vi "Test-Elevator-Set Percent.vi"() -> ()   [LabVIEW 2014, in "Comp Elevator.lvlib"]
uses:
  Comp Elevator.lvlib
  Robot Actor Framework/Trace/Trace Controller Class/Config.ctl
  Comp Motors with Encoders/Comp Motors with Encoders Class/Motor Controller Config.ctl
  Robot/Motor with Encoders/Motors with Encoders Class/Motors with Encoders Config.ctl
  Comp Motors with Encoders/Comp Motors with Encoders Class/Encoder Config.ctl
  Robot/Elevator/Elevator Class/Elevator Config.ctl
  Robot/Motor with Encoders/Motors with Encoders Class/Motors with Encoders.lvclass
  Comp Motors with Brake/Comp Motors with Brake Class/Comp Motors with Brake Config.ctl
  <vilib>/Rock Robotics/WPI/Solenoid/WPI_SolenoidChannel.ctl
  Comp Trace Controller/Comp Trace Controller Class/Comp Trace Controller.lvclass
  Comp Pressure/Comp Pressure Class/Comp Pressure.lvclass
  Robot/Elevator/Elevator Class/Elevator.lvclass
  Comp Motors with Brake/Comp Motors with Brake Class/Comp Motors with Brake.lvclass
  <vilib>/Rock Robotics/WPI/DriverStation/WPI_DriverStationRobotMode2.ctl
  Robot/Elevator/Elevator Messages/Set Rate (Percent) Msg/Set Rate (Percent) Msg.lvclass/Set Rate (Percent) Msg.ctl
  <vilib>/ActorFramework/Message Enqueuer/Message Enqueuer.lvclass/Message Enqueuer.ctl
  <vilib>/ActorFramework/Message Enqueuer/Enqueue.vi
  <vilib>/ActorFramework/Message Priority Queue/Priority Enqueue.vi
  Robot/Elevator/Elevator Messages/Set Rate (Percent) Msg/Set Rate (Percent) Msg.lvclass
  <vilib>/ActorFramework/Stop Msg/Stop Msg.lvclass
  <vilib>/ActorFramework/Actor/Actor.lvclass
  Robot Actor Framework/Trace/Trace Controller Class/Trace Controller.lvclass
  Comp Motors with Encoders/Comp Motors with Encoders Class/Comp Motors with Encoders.lvclass
panel:
  in  "Comp Motors with Brake Config":T1={"Brake Channel"=enum."Solenoid 6", "Pneumatics CAN ID"=3}
  in  "Radio Buttons":enum32{"Up", "Hold", "Down"}(radio)
  in  "Elevator Config":T3
  in  "Test Loop":u32=75
  in  "Encoder Config":T4={"P"=1.0, "D"=0.0, "F"=0.01, "I"=0.01, "Reverse Feedback Sensor"=FALSE, "Encoder Codes Per Rev"=256}
  out "Enable Tele":bool caption="Enabled Teleop"
  in  "Stop Test Loop 1":bool=TRUE
  in  "Finish Test":bool=TRUE
  in  "Start Test":bool=TRUE
  in  "Rate (Percent)":dbl(slide)=0.040816326530612165 scale=-1.0..1.0
  in  "Motos with Encoder Config":T5={"Counts  Per Revolution"=256, "Invert Encoder Direction"=FALSE, "Diameter of Revolution"=6.0, "Max RPM"=1500.0, "Encoder Control"=TRUE}
  in  "Slave Motor Controller Configs":T6[](array[typedef])
  in  "Master Motor Controller Config":T6={"Device Number"=7, "Invert Motor"=FALSE}
  in  "Trace Controller Config":T7={"Folder Pattern"="/media/sd%s1", "Starting Letter Position"=1, "Min Free Space (MB)"=50.0, "Max Folders to Check"=10, "Trace Level"=enum."Debug"} {"Min Free Space (MB)" format="%#_13g"}
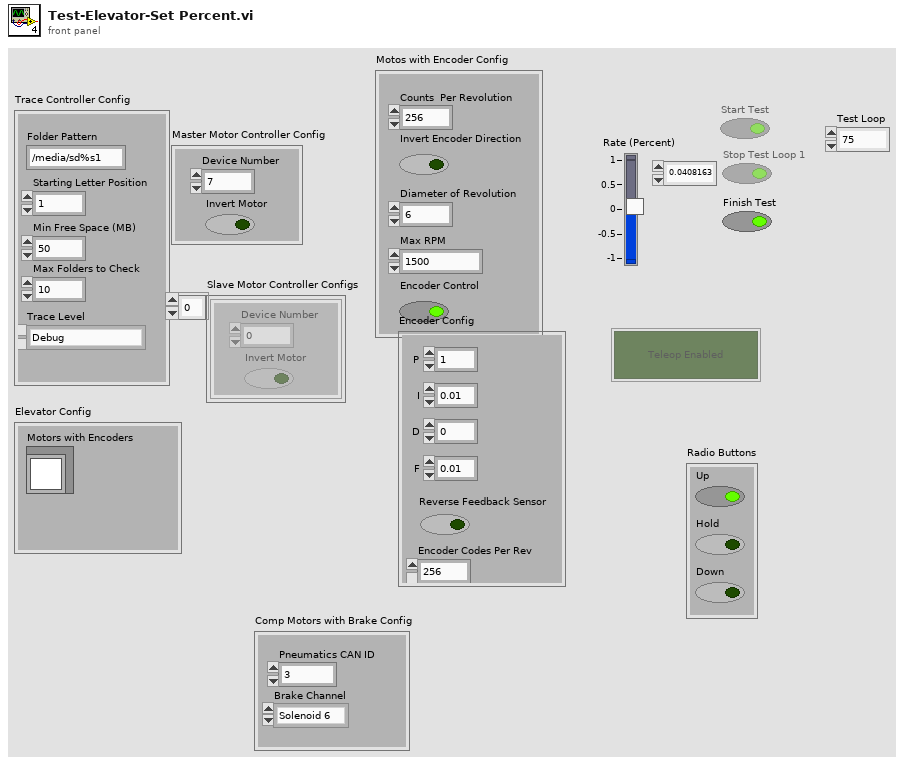
[diagram p1: front panel]
types:
  T1 = typedef "Comp Motors with Brake.lvlib/Comp Motors with Brake.lvclass/Comp Motors with Brake Config.ctl" = cluster{"Brake Channel":T2, "Pneumatics CAN ID":u8}
  T2 = typedef "WPI_SolenoidChannel.ctl" = enum8{"Solenoid 0", "Solenoid 1", "Solenoid 2", "Solenoid 3", "Solenoid 4", "Solenoid 5", "Solenoid 6", "Solenoid 7", "Invalid"}
  T3 = typedef "Elevator.lvlib/Elevator.lvclass/Elevator Config.ctl" = cluster{"Motors with Encoders ":refnum<class "Motors with Encoders.lvclass">}
  T4 = typedef "Comp Motors with Encoders.lvlib/Comp Motors with Encoders.lvclass/Encoder Config.ctl" = cluster{"P":dbl, "D":dbl, "F":dbl, "I":dbl, "Reverse Feedback Sensor":bool, "Encoder Codes Per Rev":u16}
  T5 = typedef "Motors with Encoders.lvlib/Motors with Encoders.lvclass/Motors with Encoders Config.ctl" = cluster{"Counts  Per Revolution":u32, "Invert Encoder Direction":bool, "Diameter of Revolution":dbl, "Max RPM":dbl, "Encoder Control":bool}
  T6 = typedef "Comp Motors with Encoders.lvlib/Comp Motors with Encoders.lvclass/Motor Controller Config.ctl" = cluster{"Device Number":u8, "Invert Motor":bool}
  T7 = typedef "Robot Actor Framework.lvlib/Trace.lvlib/Trace Controller.lvclass/Config.ctl" = cluster{"Folder Pattern":string, "Starting Letter Position":i32, "Min Free Space (MB)":dbl, "Max Folders to Check":u32, "Trace Level":enum16{"Critical", "Error", "Warning", "Informational", "Debug"}}
  T8 = enum16{"Critical", "Error", "Warning", "Informational", "Debug"}
  T9 = enum8{"Enabled", "Disabled", "Disabled and Grayed Out"}
  T10 = typedef "WPI_DriverStationRobotMode2.ctl" = enum16{"Autonomous Disabled", "Autonomous Enabled", "Teleop Disabled", "Teleop Enabled", "Disconnected", "Finish", "Test Disabled", "Test Enabled", "Emergency Stopped"}
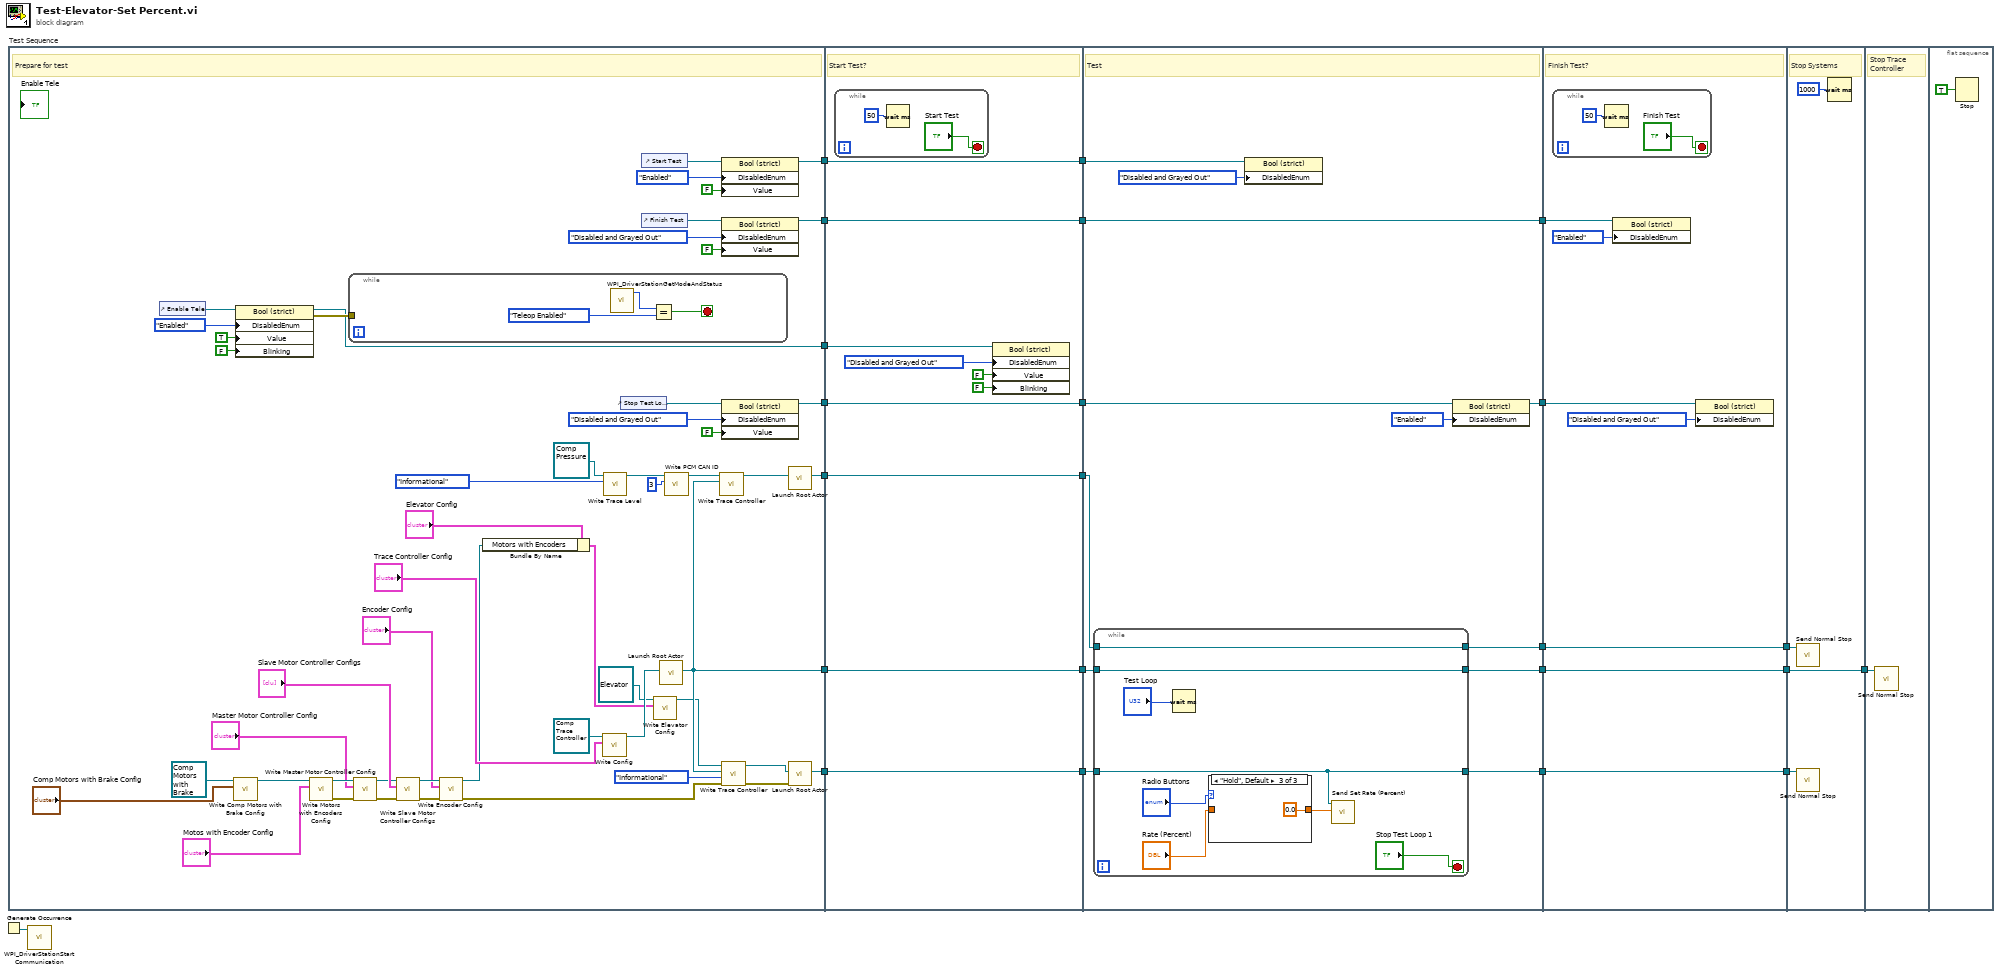
[diagram p0: block diagram]
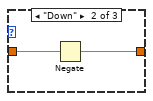
[diagram p3: hidden frame]
diagram:
  n1 = Generate Occurrence() -> (w23:refnum<k4>)
  n2 = flat-sequence "Test Sequence" {
    tunnel: [w58] -> w12
    tunnel: [w60] -> w11
    tunnel: [w59] -> w10
    tunnel: [w48] -> w9
    tunnel: [w47] -> w7
    tunnel: [w46] -> w2
    tunnel: [w40] -> w1
    tunnel: [w88] -> w15
    tunnel: [w87] -> w14
    tunnel: [w86] -> w13
    tunnel: w12 -> [w88]
    tunnel: w11 -> [w87]
    tunnel: w10 -> [w86]
    tunnel: w9 -> [w85]
    tunnel: [w85] -> w8
    tunnel: w7 -> [w84]
    tunnel: [w84] -> w6
    tunnel: [w83] -> w3
    tunnel: w2 -> [w83]
    tunnel: w1 -> [w82]
    tunnel: [w97] -> w18
    tunnel: [w99] -> w17
    tunnel: [w98] -> w16
    tunnel: w15 -> [w102]
    tunnel: w14 -> [w100]
    tunnel: w13 -> [w101]
    tunnel: w8 -> [w96]
    tunnel: w6 -> [w94]
    tunnel: [w92] -> w5
    tunnel: [w91] -> w4
    tunnel: w3 -> [w91]
    tunnel: [w121] -> w21
    tunnel: [w120] -> w20
    tunnel: [w119] -> w19
    tunnel: w18 -> [w121]
    tunnel: w17 -> [w120]
    tunnel: w16 -> [w119]
    tunnel: w5 -> [w118]
    tunnel: w4 -> [w115]
    tunnel: [w127] -> w22
    tunnel: w21 -> [w127]
    tunnel: w20 -> [w126]
    tunnel: w19 -> [w124]
    tunnel: w22 -> [w128]
    frame #0 {
      # "Prepare for test"
      n3 = control-ref of="Enable Tele"() -> (w45:refnum<vi>)
      n4 = call-dynamic "Write Comp Motors with Brake Config.vi"("Comp Motors with Brake Config"="Comp Motors with Brake Config", "Comp Motors with Brake in"=refnum<class "Comp Motors with Brake.lvclass"> refnum ("Comp Motors with Brake.lvlib:Comp Motors with Brake.lvclass")) -> ("Comp Motors with Brake out"=w25:refnum<class "Comp Motors with Brake.lvclass">)  [unwired: 8 in, 1 out]
      n5 = property class="Bool (strict)"(reference=w45, "DisabledEnum"=T9."Enabled" ("Disabled"), "Value"=TRUE, "Blinking"=FALSE) -> (reference out=w40:refnum<vi>, error out=w42:errorcluster)  [unwired: 1 in]
      n6 = call-dynamic "Write Motors with Encoders Config.vi"("Motors with Encoders Config"="Motos with Encoder Config", "Motors with Encoders in"=w25) -> ("error out"=w67:errorcluster, "Motors with Encoders out"=w33:refnum<class "Comp Motors with Brake.lvclass">)  [unwired: 8 in]
      n7 = while {
        tunnel: w42 -> [_]
        stop <- w76 stop-if-true
        n8 = call <vilib>:"WPI_DriverStationGetModeAndStatus.vi"() -> ("Robot Mode"=w78:T10)  [unwired: 10 in, 1 out]
        n9 = Equal?(x=w78, y=WPI_DriverStationRobotMode2."Teleop Enabled") -> (x = y?=w76:bool)
      }
      n10 = call-dynamic "Write Master Motor Controller Config.vi"("error in (no error)"=w67, "Master Motor Controller Config"="Master Motor Controller Config", "Comp Motors with Encoders in"=w33) -> ("error out"=w68:errorcluster, "Comp Motors with Encoders out"=w64:refnum<class "Comp Motors with Brake.lvclass">)  [unwired: 7 in]
      n11 = call-dynamic "Write Slave Motor Controller Configs.vi"("error in (no error)"=w68, "Slave Motor Controller Configs"="Slave Motor Controller Configs", "Comp Motors with Encoders in"=w64) -> ("error out"=w38:errorcluster, "Comp Motors with Encoders out"=w39:refnum<class "Comp Motors with Brake.lvclass">)  [unwired: 7 in]
      n12 = call-dynamic "Write Encoder Config.vi"("error in (no error)"=w38, "Encoder Config"="Encoder Config", "Comp Motors with Encoders in"=w39) -> ("error out"=w37:errorcluster, "Comp Motors with Encoders out"=w29:refnum<class "Comp Motors with Brake.lvclass">)  [unwired: 7 in]
      n13 = Bundle By Name(cluster="Elevator Config", "Motors with Encoders"=w29) -> (w30:T3)
      n14 = call-dynamic "Write Config.vi"("Config"="Trace Controller Config", "Trace Controller in"=refnum<class "Comp Trace Controller.lvclass"> refnum ("Comp Trace Controller.lvlib:Comp Trace Controller.lvclass")) -> ("Trace Controller out"=w63:refnum<class "Comp Trace Controller.lvclass">)  [unwired: 8 in, 1 out]
      n15 = call-dynamic "Write Trace Level.vi"("Trace Level"=T8."Informational", "System Actor in"=refnum<class "Comp Pressure.lvclass"> refnum ("Comp Pressure.lvlib:Comp Pressure.lvclass")) -> ("System Actor out"=w73:refnum<class "Comp Pressure.lvclass">)  [unwired: 8 in, 1 out]
      n16 = control-ref of="Stop Test Loop 1"() -> (w52:refnum<vi>)
      n17 = control-ref of="Start Test"() -> (w57:refnum<vi>)
      n18 = control-ref of="Finish Test"() -> (w51:refnum<vi>)
      n19 = call-dynamic "Write Elevator Config.vi"("Elevator Config"=w30, "Elevator in"=refnum<class "Elevator.lvclass"> refnum ("Elevator.lvlib:Elevator.lvclass")) -> ("Elevator out"=w27:refnum<class "Elevator.lvclass">)  [unwired: 8 in, 1 out]
      n20 = call <vilib>:"Launch Root Actor.vi"("Actor"=w63) -> ("Actor's Enqueuer"=w59:refnum<class "Message Enqueuer.lvclass">)  [unwired: 9 in, 1 out]
      n21 = call-dynamic "Write PCM CAN ID.vi"("PCM CAN ID"=u8 3, "Comp Pressure in"=w73) -> ("Comp Pressure out"=w74:refnum<class "Comp Pressure.lvclass">)  [unwired: 8 in, 1 out]
      n22 = call-dynamic "Write Trace Controller.vi"("Trace Controller"=w59, "System Actor in"=w74) -> ("System Actor out"=w75:refnum<class "Comp Pressure.lvclass">)  [unwired: 8 in, 1 out]
      n23 = property class="Bool (strict)"(reference=w57, "DisabledEnum"=T9."Enabled" ("Disabled"), "Value"=FALSE) -> (reference out=w48:refnum<vi>)  [unwired: 1 in, 1 out]
      n24 = property class="Bool (strict)"(reference=w51, "DisabledEnum"=T9."Disabled and Grayed Out" ("Disabled"), "Value"=FALSE) -> (reference out=w46:refnum<vi>)  [unwired: 1 in, 1 out]
      n25 = property class="Bool (strict)"(reference=w52, "DisabledEnum"=T9."Disabled and Grayed Out" ("Disabled"), "Value"=FALSE) -> (reference out=w47:refnum<vi>)  [unwired: 1 in, 1 out]
      n26 = call-dynamic "Write Trace Controller.vi"("error in (no error)"=w37, "Trace Level"=T8."Informational", "Trace Controller"=w59, "System Actor in"=w27) -> ("error out"=w70:errorcluster, "System Actor out"=w69:refnum<class "Elevator.lvclass">)  [unwired: 6 in]
      n27 = call <vilib>:"Launch Root Actor.vi"("Actor"=w75) -> ("Actor's Enqueuer"=w60:refnum<class "Message Enqueuer.lvclass">)  [unwired: 9 in, 1 out]
      n28 = call <vilib>:"Launch Root Actor.vi"("error in (no error)"=w70, "Actor"=w69) -> ("Actor's Enqueuer"=w58:refnum<class "Message Enqueuer.lvclass">)  [unwired: 8 in, 1 out]
    }
    frame #1 {
      # "Start Test?"
      n29 = while {
        stop <- "Start Test" stop-if-true
        n30 = Wait (ms)(milliseconds to wait=u32 50) -> ()  [unwired: 1 out]
      }
      n31 = property class="Bool (strict)"(reference=w82, "DisabledEnum"=T9."Disabled and Grayed Out" ("Disabled"), "Value"=FALSE, "Blinking"=FALSE) -> ()  [unwired: 1 in, 2 out]
    }
    frame #2 {
      # "Test"
      n32 = while {
        tunnel: w101 -> [w109]
        tunnel: [w109] -> w97
        tunnel: w102 -> [w106]
        tunnel: [w106] -> w99
        tunnel: w100 -> [w108]
        tunnel: [w108] -> w98
        stop <- "Stop Test Loop 1" stop-if-true
        n33 = Wait (ms)(milliseconds to wait="Test Loop") -> ()  [unwired: 1 out]
        n34 = case shown="\"Hold\", Default" "Radio Buttons" {
          tunnel: [w111 w112 0.0] -> w104
          tunnel: "Rate (Percent)" -> [w111 w113 _]
          frame "Up" {
          }
          frame "Down" {
            n35 = Negate(x=w113) -> (-x=w112:dbl)
          }
          frame "Hold", Default {
          }
        }
        n36 = call "Send Set Rate (Percent).vi"("Percent"=w104, "Message Enqueuer"=w106) -> ()  [unwired: 8 in, 2 out]
      }
      n37 = property class="Bool (strict)"(reference=w96, "DisabledEnum"=T9."Disabled and Grayed Out" ("Disabled")) -> ()  [unwired: 1 in, 2 out]
      n38 = property class="Bool (strict)"(reference=w94, "DisabledEnum"=T9."Enabled" ("Disabled")) -> (reference out=w92:refnum<vi>)  [unwired: 1 in, 1 out]
    }
    frame #3 {
      # "Finish Test?"
      n39 = while {
        stop <- "Finish Test" stop-if-true
        n40 = Wait (ms)(milliseconds to wait=u32 50) -> ()  [unwired: 1 out]
      }
      n41 = property class="Bool (strict)"(reference=w115, "DisabledEnum"=T9."Enabled" ("Disabled")) -> ()  [unwired: 1 in, 2 out]
      n42 = property class="Bool (strict)"(reference=w118, "DisabledEnum"=T9."Disabled and Grayed Out" ("Disabled")) -> ()  [unwired: 1 in, 2 out]
    }
    frame #4 {
      # "Stop Systems"
      n43 = call <vilib>:"Send Normal Stop.vi"("Message Enqueuer"=w124) -> ()  [unwired: 10 in, 1 out]
      n44 = call <vilib>:"Send Normal Stop.vi"("Message Enqueuer"=w126) -> ()  [unwired: 10 in, 1 out]
      n45 = Wait (ms)(milliseconds to wait=u32 1000) -> ()  [unwired: 1 out]
    }
    frame #5 {
      # "Stop Trace Controller"
      n46 = call <vilib>:"Send Normal Stop.vi"("Message Enqueuer"=w128) -> ()  [unwired: 10 in, 1 out]
    }
    frame #6 {
      n47 = Stop(stop? (T)=TRUE) -> ()
    }
  }
  n48 = call <vilib>:"WPI_DriverStationStart Communication.vi"("occurrence"=w23) -> ()  [unwired: 1 in, 10 out]
